vi "Initial State Example - Looping.vi"() -> ()   [LabVIEW 2018]
doc: "This example sends random data to your Initial State accout. To use this example first create an Initial State account for free at www.initialstate.com. Once created place your access key in the associated field and hit run."
uses:
  Controls/IS Data Point TypeDef (String).ctl
  Data Helpers/IS PolyVI Instance DBL To JSON Cluster .vi
  Data Helpers/IS PolyVI Instance Bool To JSON Cluster .vi
  Data Helpers/IS PolyVI Instance String to JSON Cluster.vi
panel:
  out "Buffer Size":i32
  in  "stop":bool
  out "Waveform Chart":dbl(graph)=0.6082396240250167
  in  "Bucket Name (Optional)":string="LabVIEW Example Bucket"
  in  "Access Key":string="FakeFakeVj0GLMeSHRkyOEAPFGhzWEmw"
  out "Response Headers":string
  out "Response Body":string
  # "Initial State Streaming LabVIEW Example"
  # "To use this example first create an Initial State account for free at www.initialstate.com. Once created place your access key in the associated field below and hit run."
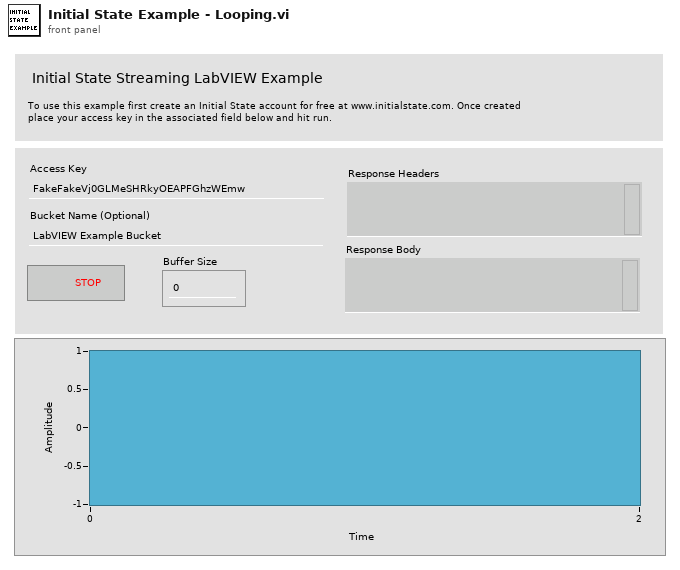
[diagram p1: front panel]
types:
  T1 = typedef "IS Data Point TypeDef (String).ctl" = cluster{"key":string, "value":string, "epoch":dbl}
  T2 = typedef "IS Session.ctl" = cluster{"Access Key":string, "HTTP Client Handle":T3}
  T3 = typedef "LabVIEWHTTPClient.lvlib/ClientHandle.ctl" = refnum<k1>
  T4 = typedef "IS Bucket Session.ctl" = cluster{"Bucket Key":string}
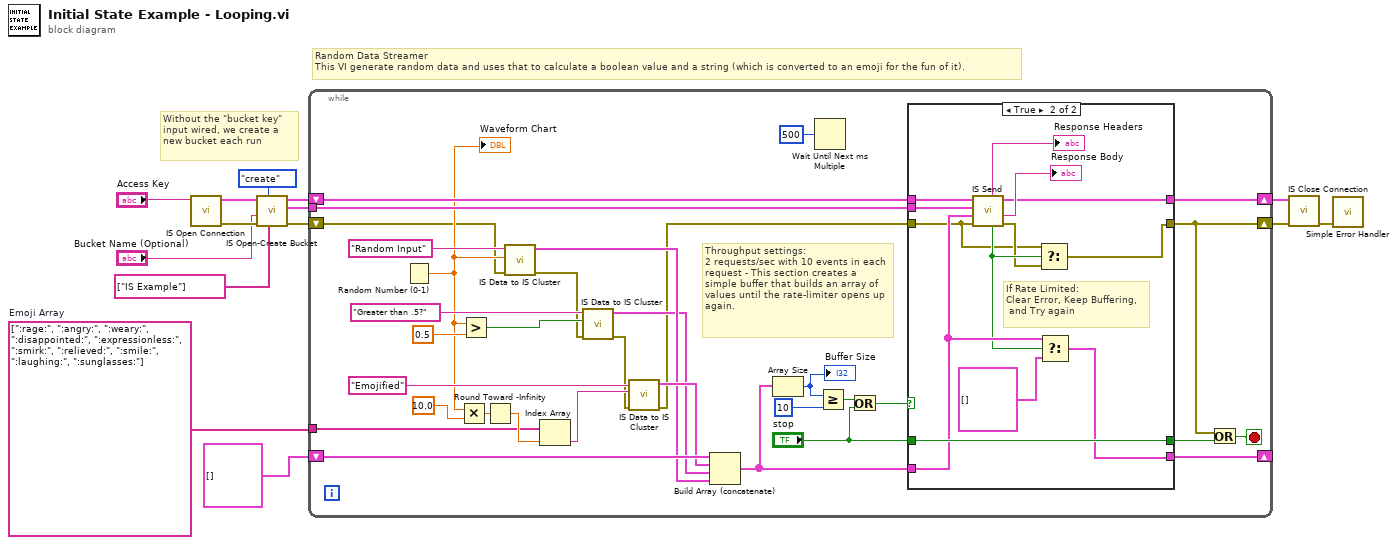
[diagram p0: block diagram]
diagram:
  w5 = string[] [":rage:", ":angry:", ":weary:", ":disappointed:", ":expressionless:", ":smirk:", ":relieved:", ":smile:", ":laughing:", ":sunglasses:"]  # Emoji Array
  # "Without the \"bucket key\" input wired, we create a new bucket each run"
  # "Random Data Streamer\nThis VI generate random data and uses that to calculate a boolean value and a string (which is converted to an emoji for the fun of it)."
  n1 = call "IS Open Connection.vi"("Access Key"="Access Key") -> ("error out"=w12:errorcluster, "IS Session"=w14:T2)  [unwired: 9 in]
  n2 = call "IS Open-Create Bucket.vi"("Tags (Optional: Auto-Populates \"labview\")"=string[] ["IS Example"] ("Tags (Optional: Auto-Populates \"labview\")"), "Operation (0: open)"=enum16{"open", "create"}."create", "error in (no error)"=w12, "Bucket Name (Optional)"="Bucket Name (Optional)", "IS Session In"=w14) -> ("error IO"=w6:errorcluster, "IS Bucket Session"=w9:T4, "IS Session Out"=w8:T2)  [unwired: 4 in]
  n3 = while {
    tunnel: w9 -> [w45]
    shift-right: [w47] -> w4
    shift-left: w8 -> [w46]
    shift-right: [w28] -> w3
    shift-left: w6 -> [w18]
    shift-right: [w43] -> _
    shift-left: T1[] [] -> [w44]
    tunnel: w5 -> [w33]
    stop <- w27 stop-if-true
    # "Throughput settings: \n2 requests/sec with 10 events in each request - This section creates a simple buffer that builds an array of values until the rate-limiter opens up again."
    n4 = Random Number (0-1)() -> (number: 0 to 1=w22:dbl)
    "Waveform Chart" <- w22
    n5 = Multiply(x=w22, y=10.0) -> (x*y=w36:dbl)
    n6 = Greater?(x=w22, y=0.5) -> (0:w21:bool)
    n7 = Round Toward -Infinity(1:w36) -> (0:w34:dbl)
    n8 = call-poly "IS Data to IS Cluster.vi"("Error In"=w18, "Stream Value"=w22, "Stream Key"="Random Input") -> ("Error Out"=w17:errorcluster, "JSON Cluster Array out"=w30:T1[])  [unwired: 7 in]
    n9 = Index Array(array=w33, index=w34) -> (element=w20:string)
    n10 = call-poly "IS Data to IS Cluster.vi"("Error In"=w17, "Stream Value"=w21, "Stream Key"="Greater than .5?") -> ("Error Out"=w16:errorcluster, "JSON Cluster Array out"=w29:T1[])  [unwired: 7 in]
    n11 = call-poly "IS Data to IS Cluster.vi"("Error In"=w16, "Stream Value"=w20, "Stream Key"="Emojified") -> ("Error Out"=w15:errorcluster, "JSON Cluster Array out"=w31:T1[])  [unwired: 7 in]
    n12 = Build Array (concatenate)(w44, w31, w29, w30) -> (w42:T1[])
    n13 = Array Size(array=w42) -> (size(s)=w41:i32)
    "Buffer Size" <- w41
    n14 = Wait Until Next ms Multiple(millisecond multiple=u32 500) -> ()  [unwired: 1 out]
    n15 = Greater Or Equal?(x=w41, y=10) -> (x >= y?=w25:bool)
    n16 = Or(x=w25, y="stop") -> (x .or. y?=w24:bool)
    n17 = case shown="True" w24 {
      tunnel: [w51 w60] -> w47
      tunnel: [w50 w52] -> w28
      tunnel: w46 -> [w51 w64]
      tunnel: w15 -> [w50 w53]
      tunnel: w45 -> [_ w63]
      tunnel: w42 -> [w49 w57]
      tunnel: [w49 w56] -> w43
      tunnel: "stop" -> [w48 w61]
      tunnel: [w48 w61] -> w26
      frame False {
      }
      frame True {
        # "If Rate Limited: \nClear Error, Keep Buffering,\n and Try again"
        n18 = call "IS Send.vi"("error in (no error)"=w53, "JSON Custer Array in"=w57, "IS Bucket Session"=w63, "IS Session in"=w64) -> ("Error out"=w54:errorcluster, "Response Body"=→"Response Body":string, "IS Session out"=w60:T2, "Rate Limit Reached?"=w55:bool, "Response Headers"=→"Response Headers":string)  [unwired: 2 in, 1 out]
        n19 = Select(t=w53, s=w55, f=w54) -> (s? t:f=w52:errorcluster)
        n20 = Select(t=w57, s=w55, f=T1[] []) -> (s? t:f=w56:T1[])
      }
    }
    n21 = Or(x=w28, y=w26) -> (x .or. y?=w27:bool)
  }
  n22 = call "IS Close Connection.vi"("error in (no error)"=w3, "IS Session In"=w4) -> ("error out"=w11:errorcluster)  [unwired: 9 in]
  n23 = call <vilib>:"Simple Error Handler.vi"("error in (no error)"=w11) -> ()  [unwired: 4 in, 5 out]
